vi "Insert Into SubPanel.vi"(8 "error in (no error)":errorcluster, 10 "SubPanel Ref":refnum<vi>, 11 "ViewableActor in":refnum<class "ViewableActor.lvclass">) -> (0 "error out":errorcluster, 3 "ViewableActor out":refnum<class "ViewableActor.lvclass">)   [LabVIEW 2012, in "Win8uiFramework.lvlib" / "ViewableActor.lvclass"]
uses:
  ViewableActor.lvclass
  ViewableActor.lvclass/ViewableActor.ctl
  Write SubPanel Ref.vi
  Read SubPanel Ref.vi
  Read UI VI Ref.vi
  <vilib>/Utility/error.llb/Simple Error Handler.vi
  Win8uiFramework.lvlib
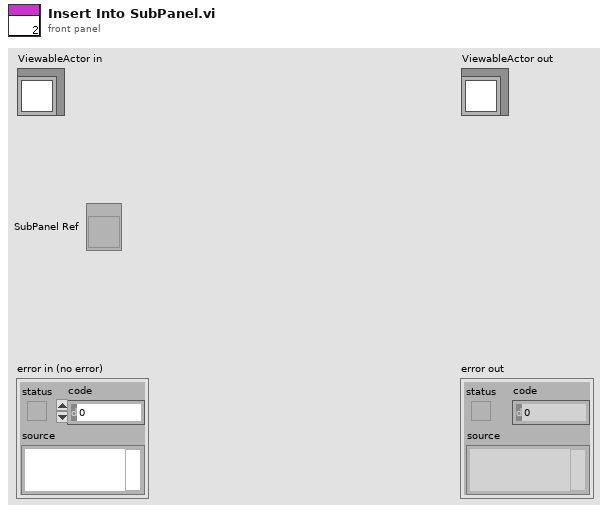
[diagram p1: front panel]
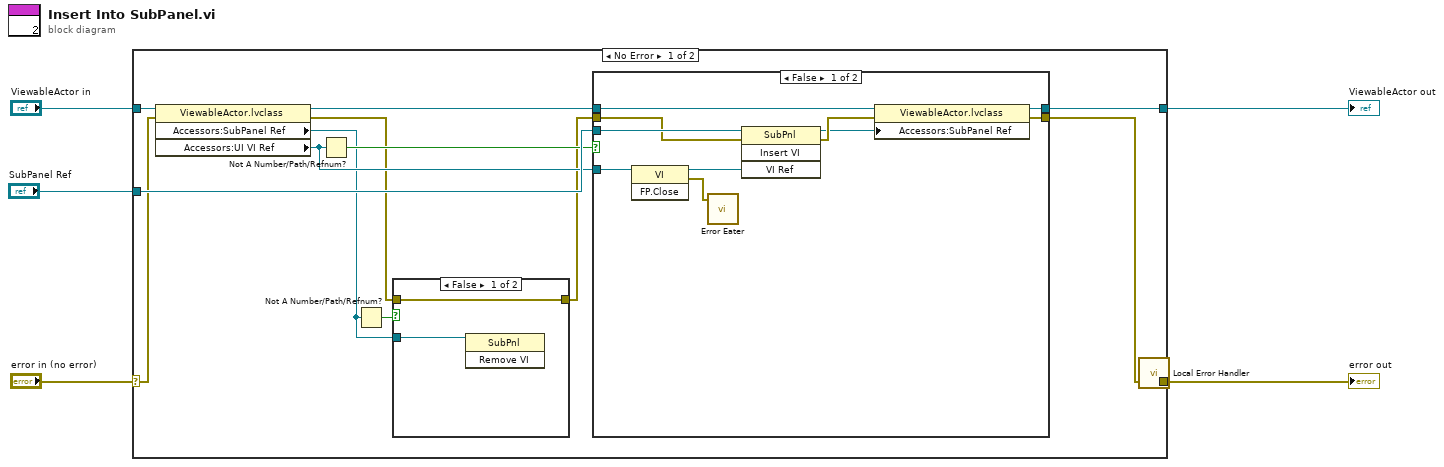
[diagram p0: block diagram]
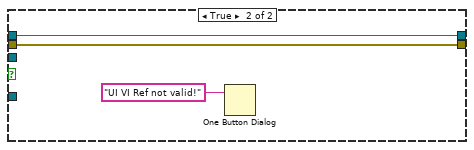
[diagram p3: hidden frame]
diagram:
  n1 = case shown="No Error" "error in (no error)" {
    selector: "error in (no error)" -> [w12 w36]
    tunnel: [w10 w36] -> w4
    tunnel: [w16 w35] -> w2
    tunnel: "ViewableActor in" -> [w18 w35]
    tunnel: "SubPanel Ref" -> [w15 _]
    frame No Error {
      n2 = property class="ViewableActor.lvclass"(reference=w18, error in=w12) -> (reference out=w17:refnum<class "ViewableActor.lvclass">, error out=w7:errorcluster, "Accessors:SubPanel Ref"=w8:refnum<vi>, "Accessors:UI VI Ref"=w13:refnum<vi>)
      n3 = Not A Number/Path/Refnum?(number/path/refnum=w13) -> (NaN/Path/Refnum?=w14:bool)
      n4 = Not A Number/Path/Refnum?(number/path/refnum=w8) -> (NaN/Path/Refnum?=w9:bool)
      n5 = case shown="False" w9 {
        tunnel: w8 -> [w20 _]
        tunnel: w7 -> [w19 w21]
        tunnel: [w19 w21] -> w6
        frame False {
          n6 = invoke on="Invoke Node" class="SubPnl" method="Remove VI"(reference=w20) -> ()  [unwired: 2 in, 3 out]
        }
        frame True {
        }
      }
      n7 = case shown="False" w14 {
        tunnel: w17 -> [w30 w33]
        tunnel: [w29 w33] -> w16
        tunnel: w15 -> [w28 _]
        tunnel: w13 -> [w22 _]
        tunnel: w6 -> [w26 w32]
        tunnel: [w25 w32] -> w11
        frame False {
          n8 = invoke class="VI" method="FP.Close"(reference=w22) -> (reference out=w31:refnum<vi>, error out=w23:errorcluster)  [unwired: 2 in, 1 out]
          n9 = call "Error Eater.vi"("error in (no error)"=w23) -> ()  [unwired: 2 in]
          n10 = invoke on="Invoke Node" class="SubPnl" method="Insert VI"(reference=w28, error in=w26, "VI Ref"=w31) -> (reference out=w24:refnum<vi>, error out=w27:errorcluster)  [unwired: 1 in, 2 out]
          n11 = property class="ViewableActor.lvclass"(reference=w30, error in=w27, "Accessors:SubPanel Ref"=w24) -> (reference out=w29:refnum<class "ViewableActor.lvclass">, error out=w25:errorcluster)
        }
        frame True {
          n12 = One Button Dialog(message="UI VI Ref not valid!") -> ()  [unwired: 1 in, 1 out]
        }
      }
      n13 = call "Local Error Handler.vi"("error in (no error)"=w11) -> ("error out"=w10:errorcluster)  [unwired: 18 in]
    }
    frame Error {
    }
  }
  "error out" <- w4
  "ViewableActor out" <- w2
